vi "DAQAsFuncGen.vi"(11 "error in":errorcluster) -> (10 "error out":errorcluster)   [LabVIEW 2025]
uses:
  <vilib>/DAQmx/write.llb/DAQmx Write (Analog 1D Wfm NChan NSamp).vi
  <vilib>/DAQmx/create/channels.llb/DAQmx Create Channel (AO-Voltage-Basic).vi
  <vilib>/DAQmx/configure/timing.llb/DAQmx Timing (Sample Clock).vi
  <vilib>/DAQmx/miscellaneous.llb/DAQmx Fill In Error Info.vi
panel:
  in  "FuncGen settings":T1={"noiseRMS"=1.0, "amplitude"=1.0, "frequency"=10.0, "signal type"=enum."Sine Wave"}
  in  "channel settings":T2={"maximum value"=10.0, "minimum value"=-10.0, "physical channels"="", "output terminal configuration"=-1, "units"=10348} {"output terminal configuration" items=["Default"=-1, "RSE"=10083, "Differential"=10106, "Pseudodifferential"=12529]; "units" items=["Volts"=10348, "From Custom Scale"=10065]}
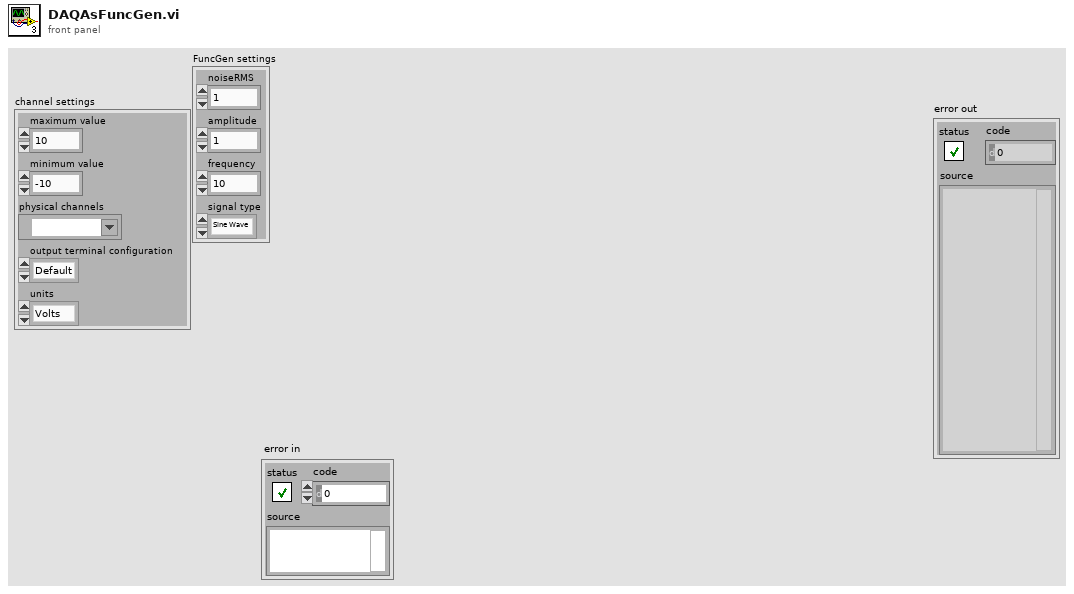
[diagram p1: front panel]
types:
  T1 = cluster{"noiseRMS":dbl, "amplitude":dbl, "frequency":dbl, "signal type":enum16{"Sine Wave", "Triangle Wave", "Square Wave", "Sawtooth Wave"}}
  T2 = cluster{"maximum value":dbl, "minimum value":dbl, "physical channels":tag, "output terminal configuration":i32, "units":i32}
  T3 = enum16{"Sine Wave", "Triangle Wave", "Square Wave", "Sawtooth Wave"}
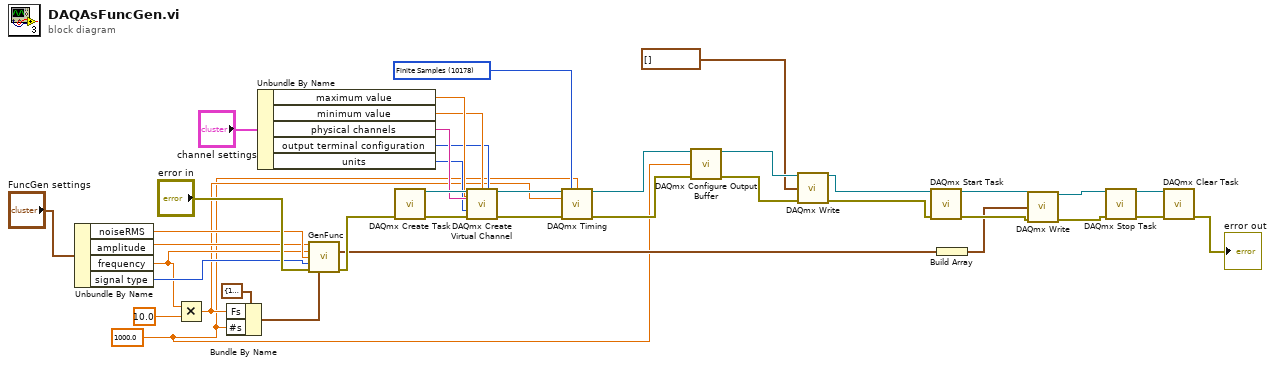
[diagram p0: block diagram]
diagram:
  w6 = 1000.0 ("#s")
  w33 = 10178 items=["Finite Samples"=10178, "Continuous Samples"=10123, "Hardware Timed Single Point"=12522] ("sample mode")
  n1 = Unbundle By Name("FuncGen settings") -> ("noiseRMS"=w17:dbl, "amplitude"=w16:dbl, "frequency"=w15:dbl, "signal type"=w18:T3)
  n2 = Multiply(x=w15, y=10.0) -> (x*y=w9:dbl)
  n3 = Bundle By Name(cluster=cluster{"Fs":dbl, "#s":dbl} {"Fs"=1000.0, "#s"=1000.0} ("sampling info"), "Fs"=w9, "#s"=w6) -> (w20:cluster{"Fs":dbl, "#s":dbl})
  n4 = Unbundle By Name("channel settings") -> ("maximum value"=w28:dbl, "minimum value"=w27:dbl, "physical channels"=w26:tag, "output terminal configuration"=w25:i32, "units"=w24:i32)
  n5 = call "GenFunc.vi"("amplitude"=w16, "frequency"=w15, "noiseRMS"=w17, "signal type"=w18, "error in (no error)"="error in", "sampling info"=w20) -> ("signal out"=w11:waveform(dbl), "error out"=w14:errorcluster)  [unwired: 8 in]
  n6 = call <vilib>:"DAQmx Create Task.vi"("error in"=w14) -> ("task out"=w32:refnum<k21>, "error out"=w36:errorcluster)  [unwired: 13 in]
  n7 = call-poly <vilib>:"DAQmx Create Virtual Channel.vi"("task in"=w32, "maximum value"=w28, "minimum value"=w27, "output terminal configuration"=w25, "physical channels"=w26, "units"=w24, "error in"=w36) -> ("task out"=w37:refnum<k21>, "error out"=w35:errorcluster)  [unwired: 7 in]
  n8 = call-poly <vilib>:"DAQmx Timing.vi"("task/channels in"=w37, "sample mode"=w33, "samples per channel"=w6, "rate"=w9, "error in"=w35) -> ("task out"=w8:refnum<k21>, "error out"=w7:errorcluster)  [unwired: 9 in]
  n9 = call <vilib>:"DAQmx Configure Output Buffer.vi"("task/channels in"=w8, "buffer size (in samples per channel)"=w6, "error in"=w7) -> ("task out"=w5:refnum<k21>, "error out"=w4:errorcluster)  [unwired: 11 in]
  n10 = call-poly <vilib>:"DAQmx Write.vi"("task/channels in"=w5, "data"=waveform(dbl)[] [], "error in"=w4) -> ("task out"=w3:refnum<k21>, "error out"=w1:errorcluster)  [unwired: 10 in, 1 out]
  n11 = call <vilib>:"DAQmx Start Task.vi"("task/channels in"=w3, "error in"=w1) -> ("task out"=w12:refnum<k21>, "error out"=w13:errorcluster)  [unwired: 12 in]
  n12 = Build Array(w11) -> (w10:waveform(dbl)[])
  n13 = call-poly <vilib>:"DAQmx Write.vi"("task/channels in"=w12, "data"=w10, "error in"=w13) -> ("task out"=w30:refnum<k21>, "error out"=w31:errorcluster)  [unwired: 10 in, 1 out]
  n14 = call <vilib>:"DAQmx Stop Task.vi"("task/channels in"=w30, "error in"=w31) -> ("task out"=w39:refnum<k21>, "error out"=w38:errorcluster)  [unwired: 12 in]
  n15 = call <vilib>:"DAQmx Clear Task.vi"("task in"=w39, "error in"=w38) -> ("error out"=→"error out":errorcluster)  [unwired: 13 in]
